vi "ParseAllBlocksMessages.vi"(11 "Path":path) -> (0 "SCM2VM Msg Cluster Array":cluster{"Names":string[], "Codes":i32[]}, 1 "VM INP from SCM Msg Cluster Array":cluster{"Names":string[], "Codes":i32[]}, 3 "VM2SCM Msg Cluster Array":cluster{"Names":string[], "Codes":i32[]}, 4 "COM2CA MSG Cluster Array":cluster{"Names":string[], "Codes":i32[]}, 5 "SCM-SCM2VP Msg Cluster Array":cluster{"Names":string[], "Codes":i32[]}, 6 "VP-SCM2VP Msg Cluster Array":cluster{"Names":string[], "Codes":i32[]}, 9 "SCM2CA Msg Cluster Array":cluster{"Names":string[], "Codes":i32[]}, 10 "CA2GUI Msg Cluster Array":cluster{"Names":string[], "Codes":i32[]}, 12 "VM2GUI Msg Cluster Array":cluster{"Names":string[], "Codes":i32[]}, 13 "VP 2 GUI Msg Cluster Array":cluster{"Names":string[], "Codes":i32[]}, 14 "VM INP from CA Msg Cluster Array":cluster{"Names":string[], "Codes":i32[]}, 15 "SCM - VM2SCM Msg Cluster Array":cluster{"Names":string[], "Codes":i32[]})   [LabVIEW 2010]
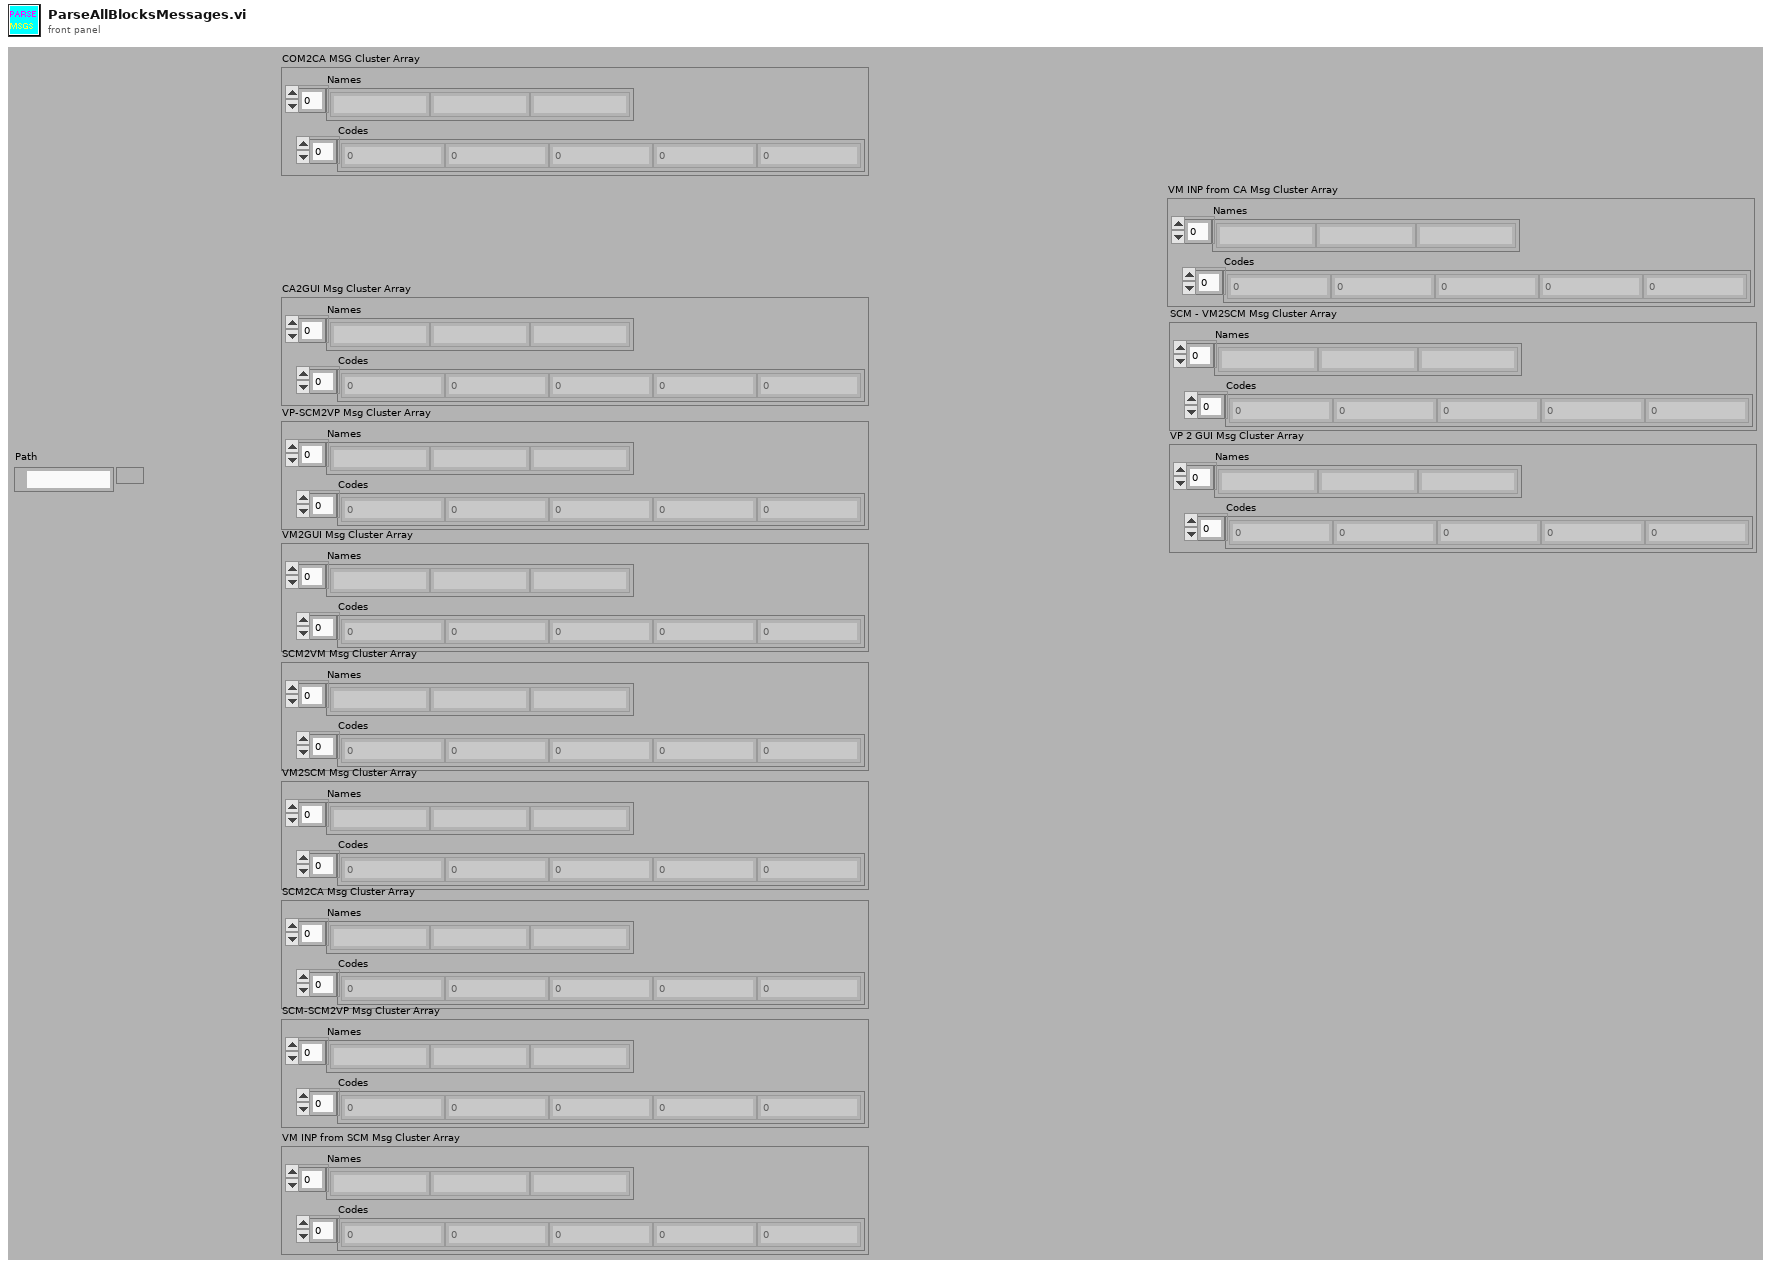
[diagram p1: front panel]
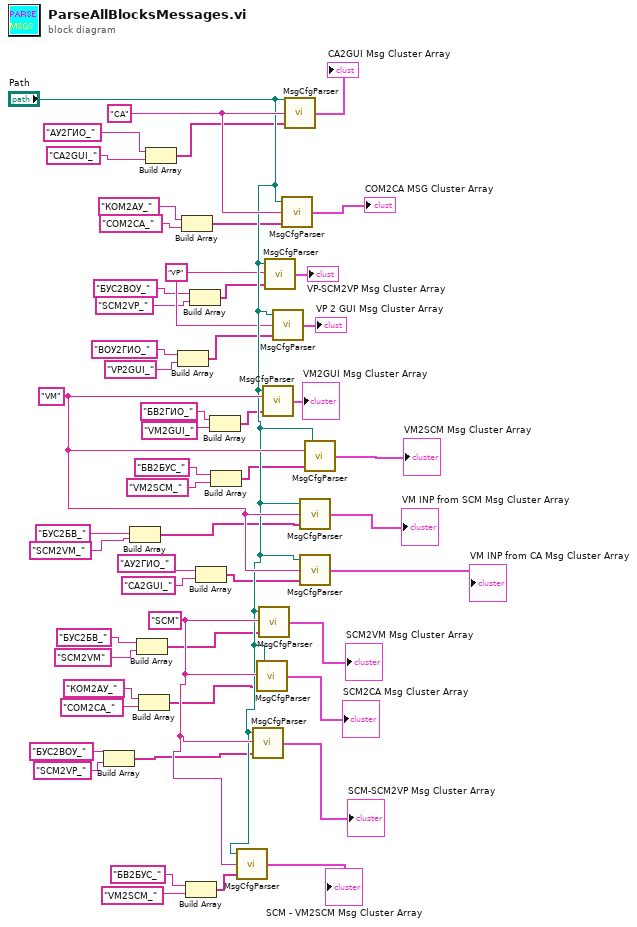
[diagram p0: block diagram]
diagram:
  w41 = "SCM" ("name or relative path")
  w43 = "VM" ("name or relative path")
  w38 = "VP" ("name or relative path")
  w52 = "CA" ("name or relative path")
  n1 = Build Array("БУС2ВОУ_" ("search string"), "SCM2VP_" ("search string")) -> (w1:string[])
  n2 = Build Array("БУС2БВ_" ("search string"), "SCM2VM_" ("search string")) -> (w8:string[])
  n3 = Build Array("БУС2БВ_" ("search string"), "SCM2VM" ("search string")) -> (w6:string[])
  n4 = Build Array("КОМ2АУ_" ("search string"), "COM2CA_" ("search string")) -> (w3:string[])
  n5 = Build Array("АУ2ГИО_" ("name or relative path"), "CA2GUI_" ("name or relative path")) -> (w34:string[])
  n6 = Build Array("ВОУ2ГИО_" ("search string"), "VP2GUI_" ("search string")) -> (w25:string[])
  n7 = Build Array("КОМ2АУ_" ("name or relative path"), "COM2CA_" ("name or relative path")) -> (w31:string[])
  n8 = Build Array("БВ2БУС_" ("search string"), "VM2SCM_" ("search string")) -> (w13:string[])
  n9 = Build Array("БУС2ВОУ_" ("search string"), "SCM2VP_" ("search string")) -> (w28:string[])
  n10 = Build Array("АУ2ГИО_" ("search string"), "CA2GUI_" ("search string")) -> (w16:string[])
  n11 = Build Array("БВ2ГИО_" ("search string"), "VM2GUI_" ("search string")) -> (w22:string[])
  n12 = Build Array("БВ2БУС_" ("search string"), "VM2SCM_" ("search string")) -> (w19:string[])
  n13 = call "MsgCfgParser.vi"("search Indexes array"=w13, "name or relative path"=w41, "stripped path"="Path") -> ("Msg Cluster Array"=→"SCM - VM2SCM Msg Cluster Array":cluster{"Names":string[], "Codes":i32[]})
  n14 = call "MsgCfgParser.vi"("search Indexes array"=w1, "name or relative path"=w41, "stripped path"="Path") -> ("Msg Cluster Array"=→"SCM-SCM2VP Msg Cluster Array":cluster{"Names":string[], "Codes":i32[]})
  n15 = call "MsgCfgParser.vi"("search Indexes array"=w3, "name or relative path"=w41, "stripped path"="Path") -> ("Msg Cluster Array"=→"SCM2CA Msg Cluster Array":cluster{"Names":string[], "Codes":i32[]})
  n16 = call "MsgCfgParser.vi"("search Indexes array"=w6, "name or relative path"=w41, "stripped path"="Path") -> ("Msg Cluster Array"=→"SCM2VM Msg Cluster Array":cluster{"Names":string[], "Codes":i32[]})
  n17 = call "MsgCfgParser.vi"("search Indexes array"=w22, "name or relative path"=w43, "stripped path"="Path") -> ("Msg Cluster Array"=→"VM2GUI Msg Cluster Array":cluster{"Names":string[], "Codes":i32[]})
  n18 = call "MsgCfgParser.vi"("search Indexes array"=w28, "name or relative path"=w38, "stripped path"="Path") -> ("Msg Cluster Array"=→"VP-SCM2VP Msg Cluster Array":cluster{"Names":string[], "Codes":i32[]})
  n19 = call "MsgCfgParser.vi"("search Indexes array"=w25, "name or relative path"=w38, "stripped path"="Path") -> ("Msg Cluster Array"=→"VP 2 GUI Msg Cluster Array":cluster{"Names":string[], "Codes":i32[]})
  n20 = call "MsgCfgParser.vi"("search Indexes array"=w31, "name or relative path"=w52, "stripped path"="Path") -> ("Msg Cluster Array"=→"COM2CA MSG Cluster Array":cluster{"Names":string[], "Codes":i32[]})
  n21 = call "MsgCfgParser.vi"("search Indexes array"=w34, "name or relative path"=w52, "stripped path"="Path") -> ("Msg Cluster Array"=→"CA2GUI Msg Cluster Array":cluster{"Names":string[], "Codes":i32[]})
  n22 = call "MsgCfgParser.vi"("search Indexes array"=w8, "name or relative path"=w43, "stripped path"="Path") -> ("Msg Cluster Array"=→"VM INP from SCM Msg Cluster Array":cluster{"Names":string[], "Codes":i32[]})
  n23 = call "MsgCfgParser.vi"("search Indexes array"=w16, "name or relative path"=w43, "stripped path"="Path") -> ("Msg Cluster Array"=→"VM INP from CA Msg Cluster Array":cluster{"Names":string[], "Codes":i32[]})
  n24 = call "MsgCfgParser.vi"("search Indexes array"=w19, "name or relative path"=w43, "stripped path"="Path") -> ("Msg Cluster Array"=→"VM2SCM Msg Cluster Array":cluster{"Names":string[], "Codes":i32[]})
